vi "Alternating LEDs.vi"() -> ()   [LabVIEW 2015]
panel:
  in  "stop":bool
  in  "Boolean":bool
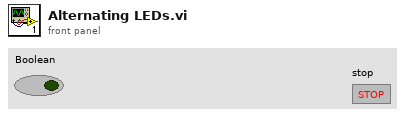
[diagram p1: front panel]
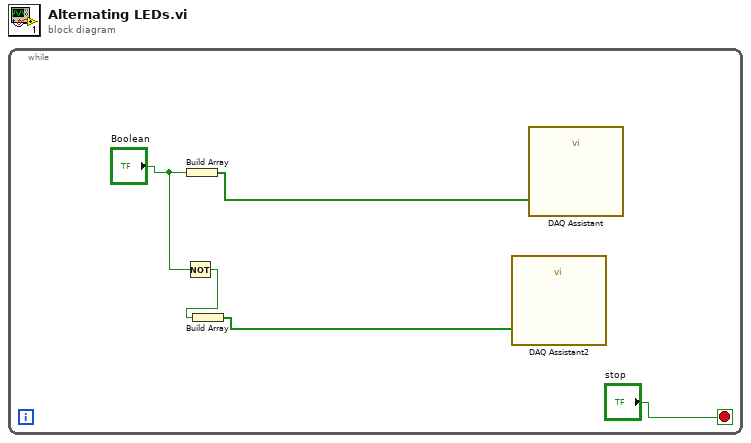
[diagram p0: block diagram]
diagram:
  n1 = while {
    stop <- "stop" stop-if-true
    n2 = Not(x="Boolean") -> (.not. x?=w1:bool)
    n3 = Build Array("Boolean") -> (w4:bool[])
    n4 = Build Array(w1) -> (w3:bool[])
    n5 = call "DAQ Assistant2"("data"=w3) -> ()  [unwired: 17 in, 2 out]
    n6 = call "DAQ Assistant"("data"=w4) -> ()  [unwired: 17 in, 2 out]
  }
